vi "onConnection.vi"(8 "error in (no error)":errorcluster, 11 "TCPConnection in":refnum<class "TCPConnection.lvclass">) -> (0 "error out":errorcluster, 3 "TCPConnection out":refnum<class "TCPConnection.lvclass">)   [LabVIEW 2013, in "MQTT_TCP.lvlib" / "TCPConnection.lvclass"]
uses:
  TCPConnection.lvclass
  MQTT_Connection/Connection/Connection.lvclass
  TCPConnection.lvclass/TCPConnection.ctl
  MQTT_Connection/Connection/Connection.lvclass/Connection.ctl
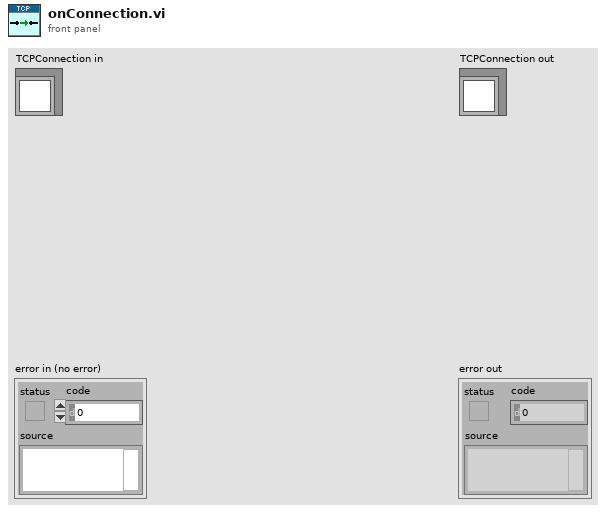
[diagram p1: front panel]
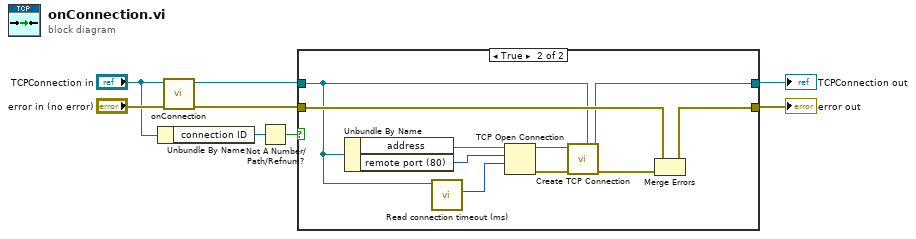
[diagram p0: block diagram]
diagram:
  n1 = Unbundle By Name("TCPConnection in") -> ("connection ID"=w1:refnum<k5>)
  n2 = call-parent "onConnection.vi"("error in (no error)"="error in (no error)", "Connection in"="TCPConnection in") -> ("error out"=w7:errorcluster, "Connection out"=w5:refnum<class "TCPConnection.lvclass">)  [unwired: 8 in]
  n3 = Not A Number/Path/Refnum?(number/path/refnum=w1) -> (NaN/Path/Refnum?=w2:bool)
  n4 = case shown="True" w2 {
    tunnel: w7 -> [w9 w15]
    tunnel: [w9 w12] -> w6
    tunnel: w5 -> [w10 w14]
    tunnel: [w10 w11] -> w4
    frame False {
    }
    frame True {
      n5 = Unbundle By Name(w14) -> ("address"=w18:string, "remote port (80)"=w17:u16)
      n6 = call "Read connection timeout (ms).vi"("Connection in"=w14) -> ("connection timeout (ms)"=w13:i32)  [unwired: 8 in, 2 out]
      n7 = TCP Open Connection(address=w18, remote port or service name=w17, timeout ms (60000)=w13) -> (connection ID=w20:refnum<k5>, error out=w19:errorcluster)  [unwired: 2 in]
      n8 = call "Create TCP Connection.vi"("TCPConnection in"=w14, "error in (no error)"=w19, "connection ID"=w20) -> ("error out"=w16:errorcluster, "TCPConnection out"=w11:refnum<class "TCPConnection.lvclass">)  [unwired: 7 in]
      n9 = Merge Errors(w15, w16) -> (w12:errorcluster)
    }
  }
  "error out" <- w6
  "TCPConnection out" <- w4
